vi "Subvi flush pixelclock.vi"(8 "Nelem":i32) -> ()   [LabVIEW 2017]
uses:
  <vilib>/rvi/Memory/Memory_Emulation/nirvimemoryFastEmulation.vi
  <vilib>/rvi/Memory/Memory_Emulation/nirvimemoryEmulation.vi
  <vilib>/rvi/Emulation/niFpgaEmulationIsFPGAContextNoSignature.vi
  <vilib>/rvi/DataTransferAndStorage/Container/Common/niFpgaContainerGetUniqueNameForEmu.vi
  <vilib>/rvi/Emulation/niFpgaProcessEmulError.vi
  <vilib>/rvi/Emulation/niFpgaSctlEmulationGetInTimedLoop.vi
  <vilib>/rvi/errors/nirviReportUnexpectedCaseInternalError (U32).vi
  <vilib>/rvi/DataTransferAndStorage/Container/XNode/niFpgaContainer.xnode
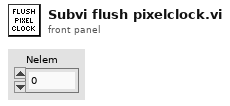
[diagram p1: front panel]
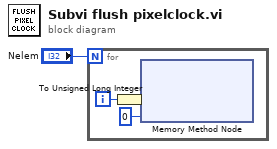
[diagram p0: block diagram]
diagram:
  n1 = for {
    N: "Nelem" -> [_]
    i -> [w4]
    n2 = To Unsigned Long Integer(number=w4) -> (unsigned 32bit integer=w2:u32)
    n3 = xnode ("Memory Method Node")("Address"=w2, "Data"=u32 0) -> ()  [unwired: 1 in, 1 out]
  }
